vi "Test XY Scanning with Alazar with bavkground subtraction.vi"() -> ()   [LabVIEW 2018]
uses:
  General/Controls/System Parameters.ctl
  General/Controls/Optical Parameters.ctl
  General/Controls/Vibratome Parameters.ctl
  General/Controls/Translation Stage Parameters.ctl
  Hardware Mfg/Thorlabs Translation Stages/Controls/Translation Stage Cluster.ctl
  General/Controls/Translation Stage Types.ctl
  General/Controls/Imaging Parameters.ctl
  General/Controls/Scan Direction.ctl
  Hardware Mfg/AlazarTech SDK/Controls/Clock Controls.ctl
  Hardware Mfg/AlazarTech SDK/Controls/Alazar Device ID.ctl
  Hardware Mfg/AlazarTech SDK/Controls/Channel Input Controls.ctl
  Hardware Mfg/AlazarTech SDK/Controls/General Trigger Settings.ctl
  Hardware Mfg/AlazarTech SDK/Controls/Trigger Engine Controls.ctl
  Hardware Mfg/AlazarTech SDK/Controls/Alazar Acquisition Settings.ctl
  General/Controls/Control cluster.ctl
  General/type defines/file type.ctl
  General/data manager action.ctl
  Hardware Mfg/AlazarTech SDK/Controls/Alazar Engine Actions.ctl
  General/Controls/Queue Manager Actions.ctl
  <vilib>/ErrorRing/Error Ring.xnode
panel:
  in  "Save?":bool
  in  "Cluster":T1={"16Bit Positions"=1000.0, "max queue size (-1, unlimited)"=-1, "File Type"=enum."image", "file path"=path "C:/Users/BoasLab/Documents/Data/Alazar data/B-line/data", "action 2"=enum."display", "#A-lines per B-line"=2048} {"16Bit Positions" min=0.0 max=10000.0 step=0.001 format="%.4f"}
  out "# elements in queue":i32
  out "Image":T4(plugin-control)
  out "# save or display":u32
  out "error out":errorcluster
  in  "Acq Settings":T5={"Window Type"=1, "Record Length"=1440, "Footer"=0, "Output Format"=11, "Offset"=0, "Records Per Buffer"=2048, "Samples per record"=2048, "Records Count (Records/Acq)"=2147483647} {"Window Type" items=["DSP_WINDOW_NONE", "DSP_WINDOW_HANNING", "DSP_WINDOW_HAMMING", "DSP_WINDOW_BLACKMAN", "DSP_WINDOW_BLACKMAN_HARRIS", "DSP_WINDOW_BARTLETT"]; "Footer" items=["FOOTER_NONE", "FOOTER_NPT"]; "Output Format" items=["FLOAT_AMP2"=10, "FLOAT_LOG"=11]}
  in  "Trigger Settings":T8={"General Trigger Settings"={"Trigger Operation"=0, "Coupling ID"=2, "Range ID"=2, "Delay"=0, "Timeout Ticks"=0, "Mode"=1, "Parameter"=1}, "Trigger Engine 1"={"Trigger Engine"=0, "Source"=2, "Slope"=1, "Level"=140}, "Trigger Engine 2"={"Trigger Engine"=1, "Source"=3, "Slope"=1, "Level"=140}} {"General Trigger Settings"."Trigger Operation" items=["J", "K", "J OR K", "J AND K", "J XOR K", "J AND NOT K", "NOT J AND K"]; "General Trigger Settings"."Coupling ID" items=["AC"=1, "DC"=2]; "General Trigger Settings"."Range ID" items=["5 V", "1 V", "TTL"]; "Trigger Engine 1"."Trigger Engine" items=["J", "K"]; "Trigger Engine 1"."Source" items=["A", "B", "External", "Disable", "C", "D"]; "Trigger Engine 1"."Slope" items=["Positive"=1, "Negative"=2]; "Trigger Engine 2"."Trigger Engine" items=["J", "K"]; "Trigger Engine 2"."Source" items=["A", "B", "External", "Disable", "C", "D"]; "Trigger Engine 2"."Slope" items=["Positive"=1, "Negative"=2]}
  in  "Ch B Input Control":T9={"Channel"=2, "Coupling"=2, "Range"=10, "Impedance"=2} {"Channel" items=["A"=1, "B"=2, "C"=4, "D"=8]; "Coupling" items=["AC"=1, "DC"=2]; "Range" items=["20 mV"=1, "40 mV"=2, "50 mV"=3, "80 mV"=4, "100 mV"=5, "200 mV"=6, "400 mV"=7, "500 mV"=8, "800 mV"=9, "1 V"=10, "1.25 V"=33, "2 V"=11, "4 V"=12, "5 V"=13, "8 V"=14, "10 V"=15, "20 V"=16]; "Impedance" items=["1 MOhm"=1, "50 Ohm"=2, ""=0]}
  in  "Ch A Input Control":T9={"Channel"=1, "Coupling"=2, "Range"=10, "Impedance"=2} {"Channel" items=["A"=1, "B"=2, "C"=4, "D"=8]; "Coupling" items=["AC"=1, "DC"=2]; "Range" items=["20 mV"=1, "40 mV"=2, "50 mV"=3, "80 mV"=4, "100 mV"=5, "200 mV"=6, "400 mV"=7, "500 mV"=8, "800 mV"=9, "1 V"=10, "1.25 V"=33, "2 V"=11, "4 V"=12, "5 V"=13, "8 V"=14, "10 V"=15, "20 V"=16]; "Impedance" items=["1 MOhm"=1, "50 Ohm"=2, ""=0]}
  in  "Device ID":T10={"System ID"=1, "Board ID"=1}
  in  "Capture Clock":T11={"Sample Rate"=100, "Decimation"=0, "Source"=2, "Edge"=0} {"Edge" items=["Rising", "Falling"]; "Source" items=["Internal"=1, "Fast External"=2, "Medium External"=3, "Slow External"=4, "External AC"=5, "External DC"=6, "External 10MHz"=7]}
  out "Acquisition":i32
  in  "stop":bool
  in  "System Parameters":T12={"Optical Parameters"={"Obj. Focal Length [mm]"=45.0, "Scan Lens EFL[mm]"=59.5, "Tube Lens EFL[mm]"=205.0, "Galvo V Range (+/-)"=10.0, "Galvo Max Half Angle [Deg]"=19.0, "Max Galvo Range[%]"=0.0}, "Vibratome"={"Z Bottom [mm]"=0.0, "Pre Cut Dwell [s]"=0.0, "Blade Frequency [RPM]"=0, "Slice Speed [mm/s]"=0.0, "Post Cut Dwell [s]"=0.0, "Ramp Time [s]"=0.0, "Start X [mm]"=0.0, "Start Y [mm]"=0.0, "Slice Length [mm]"=0.0, "Slice Axis"=enum."Y Axis", "Controller VISA Ref"="COM4"}, "Table Stages"={"X Stage"={"Position"=0.0, "Is.Enabled?"=FALSE, "Is.Connected?"=FALSE, "Device SN"="45876539", "AccelerationMaximum"=0.0, "VelocityMaximum"=0.0, "Acceleration"=0.0, "Velocity"=0.0, "waitTimeout (ms)"=0, "Model"=enum."None", "Is.Homed?"=FALSE}, "Y Stage"={"Position"=0.0, "Is.Enabled?"=FALSE, "Is.Connected?"=FALSE, "Device SN"="45876539", "AccelerationMaximum"=0.0, "VelocityMaximum"=0.0, "Acceleration"=0.0, "Velocity"=0.0, "waitTimeout (ms)"=0, "Model"=enum."None", "Is.Homed?"=FALSE}, "Z Stage"={"Position"=0.0, "Is.Enabled?"=FALSE, "Is.Connected?"=FALSE, "Device SN"="45876539", "AccelerationMaximum"=0.0, "VelocityMaximum"=0.0, "Acceleration"=0.0, "Velocity"=0.0, "waitTimeout (ms)"=0, "Model"=enum."None", "Is.Homed?"=FALSE}}, "Imaging Parameter"={"Raster Scan Direction"=enum."Uni Directional", "Pixel Dwell Time [Clock Cycles]"=1, "Flyback Time [Clock Cycles]"=200, "XY Center [um]"={"X"=1.0, "Y"=1.0}, "Pixel Step Size [um]"=2.5, "XY Image Size"=enum."2048 x 2048", "Custom"=FALSE, "Custom Size"={"X"=10, "Y"=10}, "Line Averages"=1}} {"Imaging Parameter"."Line Averages" min=1 max=30 step=1; "Imaging Parameter"."Flyback Time [Clock Cycles]" max=1000 step=1; "Imaging Parameter"."Pixel Step Size [um]" min=0.0 max=10.0 step=0.01; "Imaging Parameter"."Custom Size"."Y" min=1 max=30 step=1; "Imaging Parameter"."Custom Size"."X" min=1 max=30 step=1; "Imaging Parameter"."XY Center [um]"."Y" min=1.0 max=30.0 step=1.0; "Imaging Parameter"."XY Center [um]"."X" min=1.0 max=30.0 step=1.0; "Imaging Parameter"."Pixel Dwell Time [Clock Cycles]" max=10 step=1}
  in  "Galvo HW Parameters":T20={"Analog Out Channel"="GalvoCtrl/ao0,GalvoCtrl/ao1", "Min Voltage"=-10.0, "Max Voltage"=10.0, "Pixel Clock Source"="/GalvoCtrl/PFI0", "Sample Rate"=1000.0, "Line Clock Out Ch"="GalvoCtrl/port0/line0"}
  # "X"
  # "X"
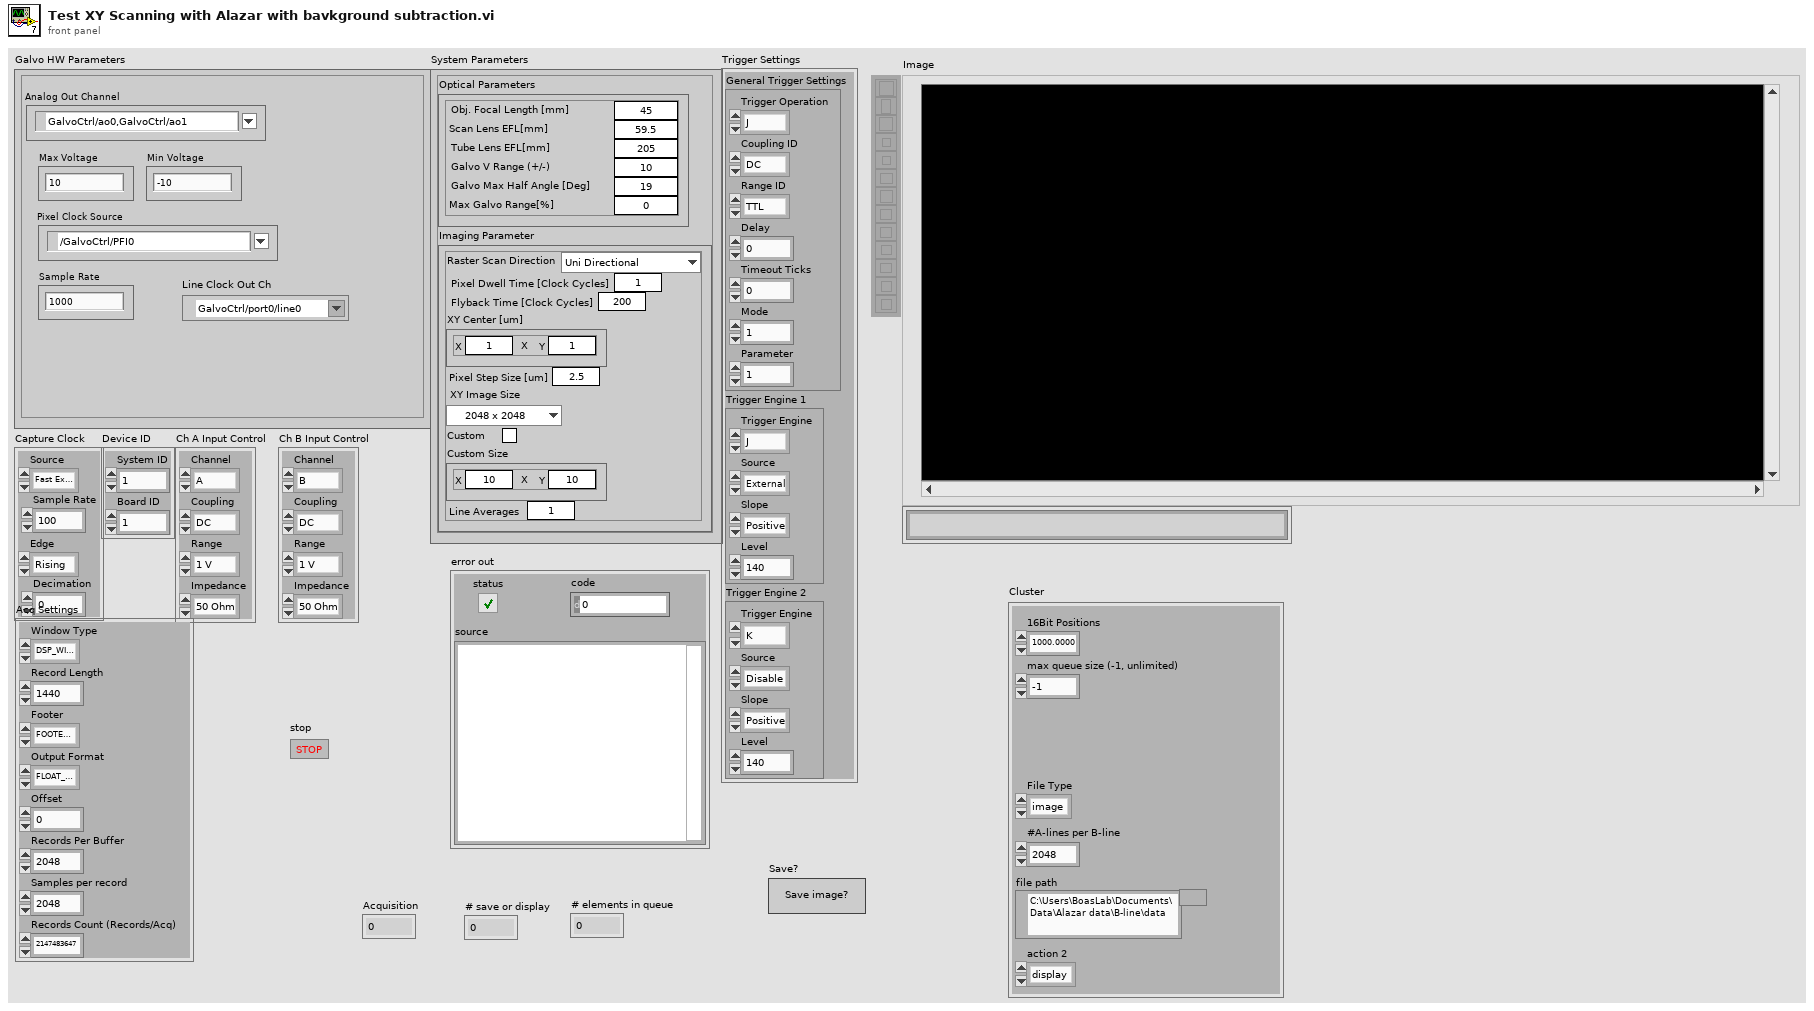
[diagram p1: front panel]
types:
  T1 = typedef "Control cluster.ctl" = cluster{"16Bit Positions":dbl, "max queue size (-1, unlimited)":i32, "File Type":T2, "file path":path, "action 2":T3, "#A-lines per B-line":u32}
  T2 = typedef "file type.ctl" = enum16{"text", "image", "binary"}
  T3 = typedef "data manager action.ctl" = enum16{"Init", "save as text", "Uninit", "open file", "close file", "display", "display and Save"}
  T4 = typedef "IMAQ Image.ctl" = refnum<image>
  T5 = typedef "Alazar Acquisition Settings.ctl" = cluster{"Window Type":u32, "Record Length":u32, "Footer":u32, "Output Format":u32, "Offset":u32, "Records Per Buffer":u32, "Samples per record":u32, "Records Count (Records/Acq)":u32}
  T6 = typedef "General Trigger Settings.ctl" = cluster{"Trigger Operation":u32, "Coupling ID":u32, "Range ID":u32, "Delay":u32, "Timeout Ticks":u32, "Mode":u32, "Parameter":u32}
  T7 = typedef "Trigger Engine Controls.ctl" = cluster{"Trigger Engine":u32, "Source":u32, "Slope":u32, "Level":u32}
  T8 = cluster{"General Trigger Settings":T6, "Trigger Engine 1":T7, "Trigger Engine 2":T7}
  T9 = typedef "Channel Input Controls.ctl" = cluster{"Channel":u8, "Coupling":u32, "Range":u32, "Impedance":u32}
  T10 = typedef "Alazar Device ID.ctl" = cluster{"System ID":u32, "Board ID":u32}
  T11 = typedef "Clock Controls.ctl" = cluster{"Sample Rate":u32, "Decimation":u32, "Source":u32, "Edge":u32}
  T12 = typedef "System Parameters.ctl" = cluster{"Optical Parameters":T13, "Vibratome":T14, "Table Stages":T15, "Imaging Parameter":T18}
  T13 = typedef "Optical Parameters.ctl" = cluster{"Obj. Focal Length [mm]":dbl, "Scan Lens EFL[mm]":dbl, "Tube Lens EFL[mm]":dbl, "Galvo V Range (+/-)":dbl, "Galvo Max Half Angle [Deg]":dbl, "Max Galvo Range[%]":dbl}
  T14 = typedef "Vibratome Parameters.ctl" = cluster{"Z Bottom [mm]":dbl, "Pre Cut Dwell [s]":dbl, "Blade Frequency [RPM]":u16, "Slice Speed [mm/s]":dbl, "Post Cut Dwell [s]":dbl, "Ramp Time [s]":dbl, "Start X [mm]":dbl, "Start Y [mm]":dbl, "Slice Length [mm]":dbl, "Slice Axis":enum16{"X Axis", "Y Axis", "Z Axis"}, "Controller VISA Ref":refnum<visa-resource-name>}
  T15 = typedef "Translation Stage Parameters.ctl" = cluster{"X Stage":T16, "Y Stage":T16, "Z Stage":T16}
  T16 = typedef "Translation Stage Cluster.ctl" = cluster{"Position":dbl, "Is.Enabled?":bool, "Is.Connected?":bool, "Device SN":string, "AccelerationMaximum":dbl, "VelocityMaximum":dbl, "Acceleration":dbl, "Velocity":dbl, "waitTimeout (ms)":i32, "Model":T17, "Is.Homed?":bool}
  T17 = typedef "Translation Stage Types.ctl" = enum16{"None", "Thorlabs LTS", "Thorlabs MLJ"}
  T18 = typedef "Imaging Parameters.ctl" = cluster{"Raster Scan Direction":T19, "Pixel Dwell Time [Clock Cycles]":u16, "Flyback Time [Clock Cycles]":u16, "XY Center [um]":cluster{"X":dbl, "Y":dbl}, "Pixel Step Size [um]":dbl, "XY Image Size":enum16{"32 x 32", "64 x 64", "128 x 128", "256 x 256", "512 x 512", "1024 x 1024", "2048 x 2048"}, "Custom":bool, "Custom Size":cluster{"X":u16, "Y":u16}, "Line Averages":u8}
  T19 = typedef "Scan Direction.ctl" = enum16{"Uni Directional", "Bi Directional", "None"}
  T20 = cluster{"Analog Out Channel":tag, "Min Voltage":dbl, "Max Voltage":dbl, "Pixel Clock Source":tag, "Sample Rate":dbl, "Line Clock Out Ch":tag}
  T21 = typedef "Queue Manager Actions.ctl" = enum16{"Init", "Enqueue", "Enqueue All", "Preview Queue", "Dequeue", "Get Status", "Flush Queue", "Flush All Queues", "Release All Queues", "Release Queue", "Enqueue at Opposite End"}
  T22 = typedef "Alazar Engine Actions.ctl" = enum16{"Init", "Config Clock", "Config Ch", "Config Trig", "Config Non-FFT Acq.", "Non-FFT Acquire", "Load background from Non-FFT buffer", "enable background subtrac", "disable background subtrac", "load background from file", "load background from elsewhere", "start acquire", "background subtraction", "Config Acq.", "Acquire", "UnInit"}
  T23 = enum16{"Init", "Calc & Write Scan Pattern", "Start Galvo Task", "Is Task Done?", "Stop Galvo", "Uninit"}
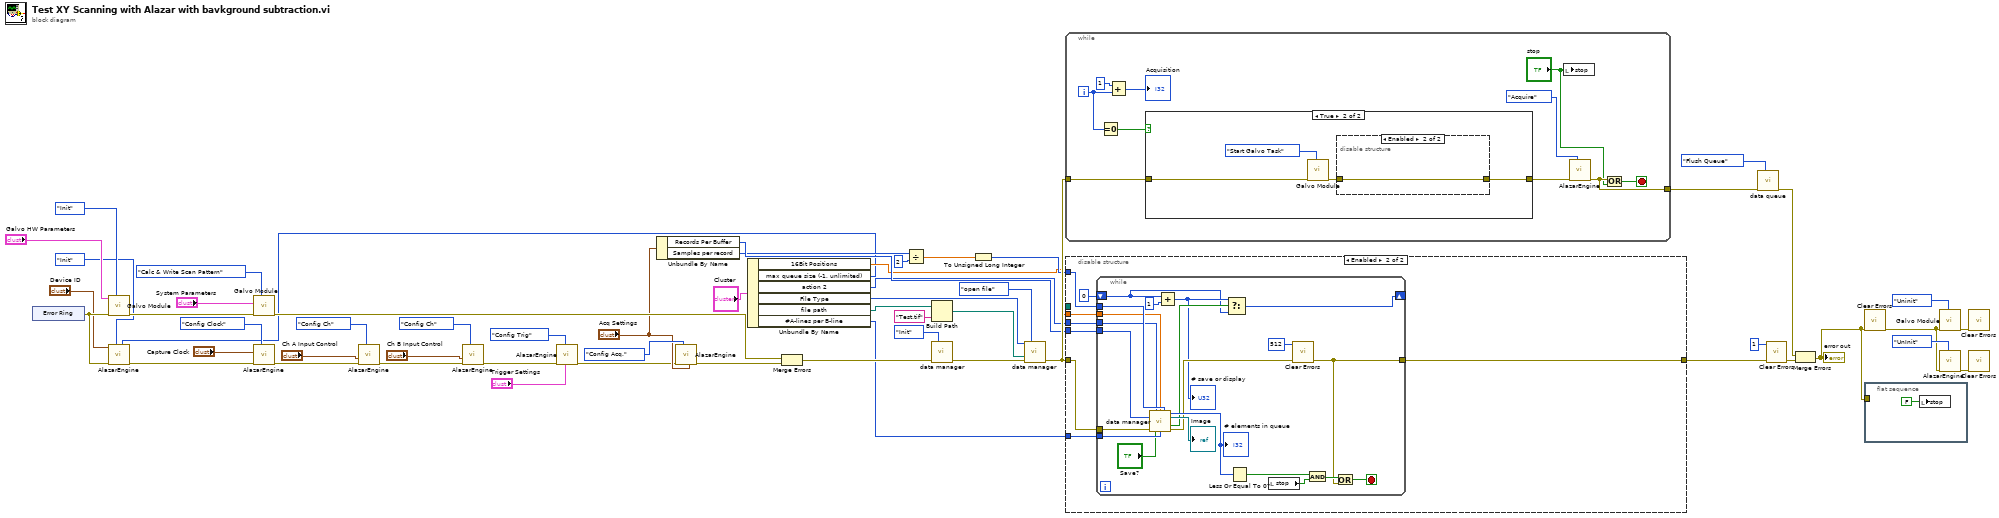
[diagram p0: block diagram]
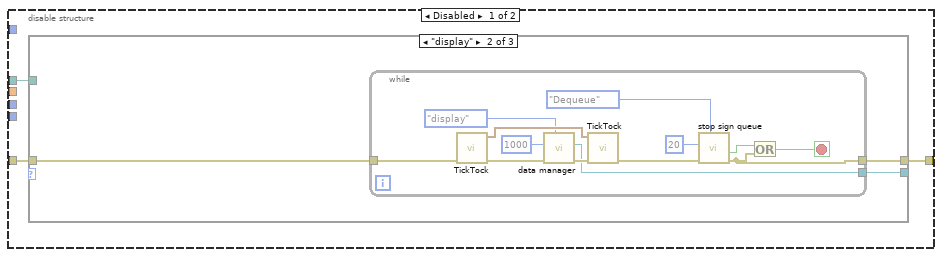
[diagram p2: hidden frame]
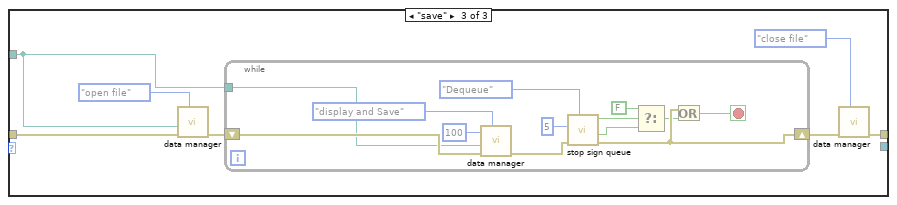
[diagram p4: hidden frame]
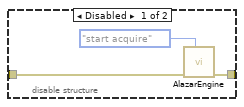
[diagram p6: hidden frame]
diagram:
  n1 = xnode "Error Ring"() -> ("error out"=w47:errorcluster)
  n2 = call "Galvo Module.vi"("Action"=T23."Init", "error in (no error)"=w47, "Galvo HW Parameters"="Galvo HW Parameters") -> ("error out"=w54:errorcluster)  [unwired: 7 in, 1 out]
  n3 = call "Galvo Module.vi"("Action"=T23."Calc & Write Scan Pattern", "error in (no error)"=w54, "System Parameters"="System Parameters") -> ("error out"=w53:errorcluster)  [unwired: 7 in, 1 out]
  n4 = Unbundle By Name("Acq Settings") -> ("Records Per Buffer"=w14:u32, "Samples per record"=w11:u32)
  n5 = Unbundle By Name("Cluster") -> ("16Bit Positions"=w3:dbl, "max queue size (-1, unlimited)"=w2:i32, "action 2"=w5:T3, "File Type"=w4:T2, "file path"=w6:path, "#A-lines per B-line"=w1:u32)
  n6 = call "AlazarEngine.vi"("max queue size (-1, unlimited)"=w2, "Action"=Alazar_Engine_Actions."Init", "error in (no error)"=w47, "Device ID"="Device ID") -> ("error out"=w50:errorcluster)  [unwired: 5 in, 2 out]
  n7 = call "AlazarEngine.vi"("Action"=Alazar_Engine_Actions."Config Clock", "error in (no error)"=w50, "Capture Clock"="Capture Clock") -> ("error out"=w49:errorcluster)  [unwired: 6 in, 2 out]
  n8 = call "AlazarEngine.vi"("Action"=Alazar_Engine_Actions."Config Ch", "error in (no error)"=w49, "Ch Input Control"="Ch A Input Control") -> ("error out"=w48:errorcluster)  [unwired: 6 in, 2 out]
  n9 = call "AlazarEngine.vi"("Action"=Alazar_Engine_Actions."Config Ch", "error in (no error)"=w48, "Ch Input Control"="Ch B Input Control") -> ("error out"=w38:errorcluster)  [unwired: 6 in, 2 out]
  n10 = call "AlazarEngine.vi"("Trigger Settings"="Trigger Settings", "Action"=Alazar_Engine_Actions."Config Trig", "error in (no error)"=w38) -> ("error out"=w15:errorcluster)  [unwired: 6 in, 2 out]
  n11 = call "AlazarEngine.vi"("Acq Settings"="Acq Settings", "Action"=Alazar_Engine_Actions."Config Acq.", "error in (no error)"=w15) -> ("error out"=w34:errorcluster)  [unwired: 6 in, 2 out]
  n12 = Merge Errors(w53, w34) -> (w28:errorcluster)
  n13 = Divide(x=w11, y=u32 2) -> (x/y=w9:dbl)
  n14 = Build Path(base path=w6, name or relative path="Test.tif") -> (appended path=w19:path)
  n15 = call "data manager.vi"("action"=data_manager_action."Init", "error in (no error)"=w28) -> ("error out"=w24:errorcluster)  [unwired: 10 in, 3 out]
  n16 = To Unsigned Long Integer(number=w9) -> (unsigned 32bit integer=w8:u32)
  n17 = call "data manager.vi"("File Type"=w4, "action"=data_manager_action."open file", "file (use dialog)"=w19, "error in (no error)"=w24) -> ("error out"=w22:errorcluster)  [unwired: 8 in, 3 out]
  n18 = while {
    tunnel: w22 -> [w66]
    tunnel: [w62] -> w16
    i -> [w59]
    stop <- w61 stop-if-true
    n19 = Equal To 0?(x=w59) -> (x = 0?=w65:bool)
    n20 = Add(x=1, y=w59) -> (x+y=→"Acquisition":i32)
    n21 = case shown="True" w65 {
      tunnel: w66 -> [w67 w71]
      tunnel: [w67 w68] -> w64
      frame False {
      }
      frame True {
        n22 = call "Galvo Module.vi"("Action"=T23."Start Galvo Task", "error in (no error)"=w71) -> ("error out"=w69:errorcluster)  [unwired: 8 in, 1 out]
        n23 = disable-structure shown="Enabled" {
          disable-tunnel: w69 -> [w74 w75]
          disable-tunnel: [w73 w75] -> w68
          frame Disabled {
            n24 = call "AlazarEngine.vi"("Action"=Alazar_Engine_Actions."start acquire", "error in (no error)"=w74) -> ("error out"=w73:errorcluster)  [unwired: 7 in, 2 out]
          }
          frame Enabled {
          }
        }
      }
    }
    n25 = local write "stop"("stop") -> ()
    n26 = call "AlazarEngine.vi"("Action"=Alazar_Engine_Actions."Acquire", "error in (no error)"=w64) -> ("error out"=w62:errorcluster)  [unwired: 7 in, 2 out]
    n27 = Or(x=w62, y="stop") -> (x .or. y?=w61:bool)
  }
  n28 = disable-structure shown="Enabled" {
    disable-tunnel: w22 -> [w79 w126]
    disable-tunnel: [w77 w125] -> w27
    disable-tunnel: w14 -> [_ w124]
    disable-tunnel: _ -> [w76 _]
    disable-tunnel: w8 -> [_ w122]
    disable-tunnel: w5 -> [_ w121]
    disable-tunnel: w3 -> [_ w120]
    disable-tunnel: w1 -> [_ w119]
    frame Disabled {
      n29 = case shown="\"display\"" w78 {
        tunnel: w79 -> [w80 w83 w102]
        tunnel: [w80 w82 w99] -> w77
        tunnel: [_ w81 _] -> _
        tunnel: w76 -> [_ _ w98]
        frame Default {
        }
        frame "display" {
          n30 = while {
            tunnel: w83 -> [w95]
            tunnel: [w96] -> w82
            tunnel: [w84] -> w81
            stop <- w97 stop-if-true
            n31 = call "TickTock.vi"("Error In"=w95) -> ("Error Out"=w91:errorcluster, "Current Time (Out)"=w88:timestamp)  [unwired: 8 in, 1 out]
            n32 = call "data manager.vi"("action"=data_manager_action."display", "error in (no error)"=w91, "# B-lines"=1000 ("timeout in ms (-1)")) -> ("error out"=w90:errorcluster, "Image"=w84:T4)  [unwired: 5 in, 2 out]
            n33 = call "TickTock.vi"("Error In"=w90, "Current Time (In)"=w88) -> ("Error Out"=w89:errorcluster, "dt"=w86:dbl)  [unwired: 7 in, 1 out]
            n34 = call "stop sign queue.vi"("Action"=Queue_Manager_Actions."Dequeue", "error in (no error)"=w89, "time out"=20) -> ("error out"=w96:errorcluster, "stop out"=w93:bool)  [unwired: 5 in, 2 out]
            n35 = Or(x=w93, y=w96) -> (x .or. y?=w97:bool)
          }
        }
        frame "save" {
          n36 = call "data manager.vi"("action"=data_manager_action."open file", "error in (no error)"=w102, "file (use dialog)"=w98) -> ("error out"=w101:errorcluster)  [unwired: 5 in, 3 out]
          n37 = while {
            shift-right: [w113] -> w100
            shift-left: w101 -> [w118]
            tunnel: w98 -> [w106]
            stop <- w116 stop-if-true
            n38 = call "data manager.vi"("action"=data_manager_action."display and Save", "error in (no error)"=w118, "file (use dialog)"=w106, "# B-lines"=100 ("timeout in ms (-1)")) -> ("error out"=w114:errorcluster, "File Type"=w115:T2)  [unwired: 3 in, 3 out]
            n39 = call "stop sign queue.vi"("Action"=Queue_Manager_Actions."Dequeue", "error in (no error)"=w114, "time out"=5) -> ("error out"=w113:errorcluster, "stop out"=w108:bool, "timed out?"=w110:bool)  [unwired: 5 in, 1 out]
            n40 = Select(t=FALSE, s=w110, f=w108) -> (s? t:f=w107:bool)
            n41 = Or(x=w113, y=w107) -> (x .or. y?=w116:bool)
          }
          n42 = call "data manager.vi"("action"=data_manager_action."close file", "error in (no error)"=w100) -> ("error out"=w99:errorcluster)  [unwired: 6 in, 3 out]
        }
      }
    }
    frame Enabled {
      n43 = while {
        tunnel: w126 -> [w147]
        tunnel: [w140] -> w125
        tunnel: w124 -> [w132]
        shift-right: [w134] -> _
        shift-left: 0 -> [w133]
        tunnel: w122 -> [w131]
        tunnel: w121 -> [w130]
        tunnel: w120 -> [w129]
        tunnel: w119 -> [w128]
        stop <- w146 stop-if-true
        n44 = call "data manager.vi"("action"=w130, "16Bit Positions"=w129, "Z pixels"=w131, "# B-lines"=w132, "error in (no error)"=w147, "Save?"="Save?", "#A-lines per B-line"=w128) -> ("# elements in queue"=w145:i32, "Image"=→"Image":T4, "non empty buffer?"=w137:bool, "error out"=w141:errorcluster)  [unwired: 5 in]
        "# elements in queue" <- w145
        n45 = Add(x=w133, y=u32 1) -> (x+y=w135:u32)
        "# save or display" <- w135
        n46 = Select(t=w135, s=w137, f=w133) -> (s? t:f=w134:u32)
        n47 = Less Or Equal To 0?(x=w145) -> (x <= 0?=w144:bool)
        n48 = local read "stop"() -> (w138:bool)
        n49 = call <vilib>:"Clear Errors.vi"("error in (no error)"=w141, "specific error code to clear (0: all)"=512) -> ("error out"=w140:errorcluster)  [unwired: 4 in, 1 out]
        n50 = And(x=w144, y=w138) -> (x .and. y?=w143:bool)
        n51 = Or(x=w143, y=w140) -> (x .or. y?=w146:bool)
      }
    }
  }
  n52 = call "data queue.vi"("Action"=Queue_Manager_Actions."Flush Queue", "error in (no error)"=w16) -> ("error out"=w13:errorcluster)  [unwired: 6 in, 3 out]
  n53 = call <vilib>:"Clear Errors.vi"("error in (no error)"=w27, "specific error code to clear (0: all)"=1) -> ("error out"=w26:errorcluster)  [unwired: 4 in, 1 out]
  n54 = Merge Errors(w13, w26) -> (w18:errorcluster)
  "error out" <- w18
  n55 = call <vilib>:"Clear Errors.vi"("error in (no error)"=w18) -> ("error out"=w31:errorcluster)  [unwired: 5 in, 1 out]
  n56 = flat-sequence {
    tunnel: w18 -> [_]
    frame #0 {
      n57 = local write "stop"(FALSE ("stop")) -> ()
    }
  }
  n58 = call "Galvo Module.vi"("Action"=T23."Uninit", "error in (no error)"=w31) -> ("error out"=w30:errorcluster)  [unwired: 8 in, 1 out]
  n59 = call "AlazarEngine.vi"("Action"=Alazar_Engine_Actions."UnInit", "error in (no error)"=w31) -> ("error out"=w29:errorcluster)  [unwired: 7 in, 2 out]
  n60 = call <vilib>:"Clear Errors.vi"("error in (no error)"=w30) -> ()  [unwired: 5 in, 2 out]
  n61 = call <vilib>:"Clear Errors.vi"("error in (no error)"=w29) -> ()  [unwired: 5 in, 2 out]
